vi "UMLEditor_SetMouseCursor.vi"(7 "ViRefToActOn":refnum<vi>, 8 "error in (no error)":errorcluster, 11 "CursorType":T1=enum."NS") -> (0 "error out":errorcluster, 3 "AllCursors":refnum<k1>[](array[refnum]))   [LabVIEW 2016]
uses:
  <resource>/Framework/Providers/Open_GDS/UML/UMLEditor/UMLEditor_Cursortype.ctl
  <vilib>/Utility/cursorutil.llb/Set Cursor (Icon Pict).vi
  <vilib>/Utility/cursorutil.llb/Set Cursor (Cursor ID).vi
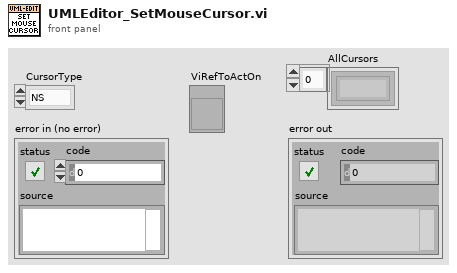
[diagram p1: front panel]
types:
  T1 = typedef "UMLEditor_Cursortype.ctl" = enum16{"Arrow", "Move", "Finger", "Wait", "NS", "WE", "NESW", "NWSE"}
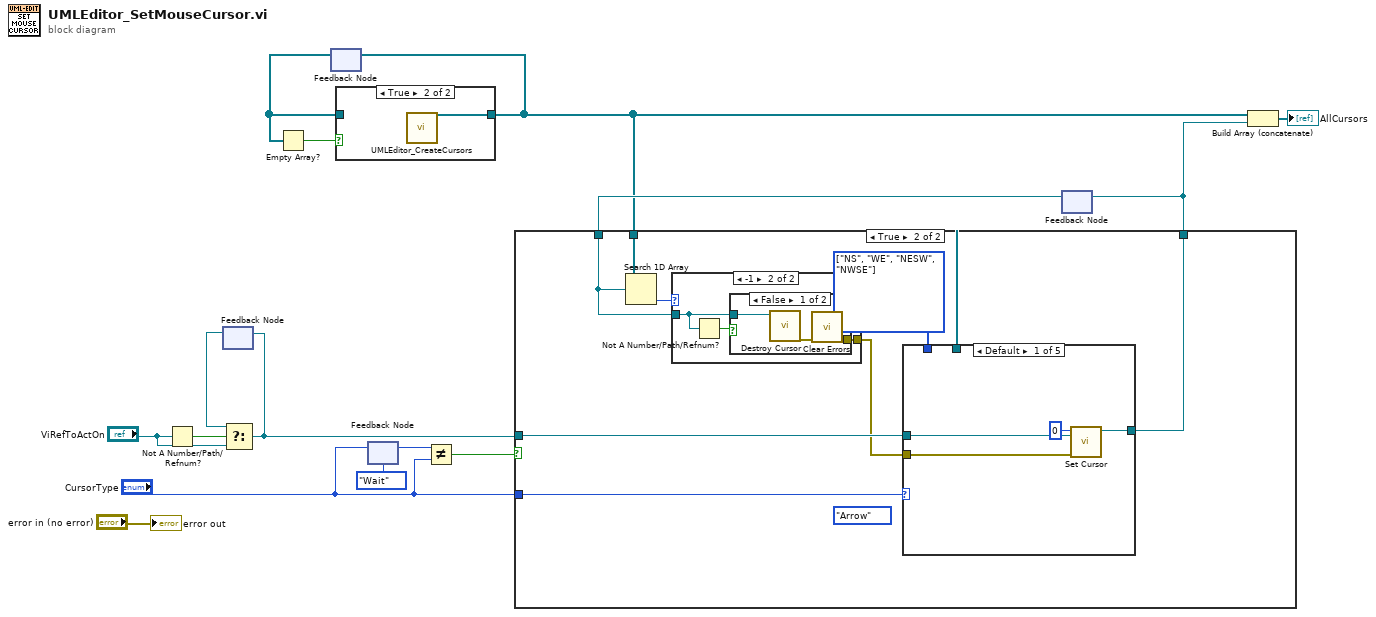
[diagram p0: block diagram]
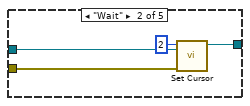
[diagram p3: hidden frame]
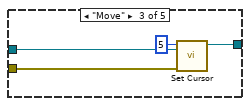
[diagram p4: hidden frame]
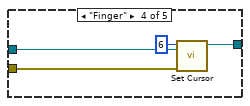
[diagram p5: hidden frame]
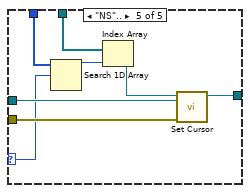
[diagram p6: hidden frame]
diagram:
  n1 = Not A Number/Path/Refnum?(number/path/refnum="ViRefToActOn") -> (NaN/Path/Refnum?=w13:bool)
  n2 = feedback #1() -> (w11:refnum<vi>)  [unwired: 1 in]
  n3 = Select(t=w11, s=w13, f="ViRefToActOn") -> (s? t:f=w10:refnum<vi>)
  n4 = feedback-in #1(w10) -> ()
  n5 = feedback #2() -> (w14:refnum<k1>[])  [unwired: 1 in]
  n6 = Empty Array?(array=w14) -> (empty?=w15:bool)
  n7 = case shown="True" w15 {
    tunnel: w14 -> [w16 _]
    tunnel: [w16 w17] -> w2
    frame False {
    }
    frame True {
      n8 = call <resource>:"UMLEditor_CreateCursors.vi"() -> ("Array"=w17:refnum<k1>[])  [unwired: 10 in, 1 out]
    }
  }
  n9 = feedback-in #2(w2) -> ()
  n10 = feedback #3(UMLEditor_Cursortype."Wait" ("CursorType")) -> (w4:T1)
  n11 = feedback-in #3("CursorType") -> ()
  n12 = Not Equal?(x=w4, y="CursorType") -> (x != y?=w1:bool)
  n13 = feedback #4() -> (w9:refnum<k1>)  [unwired: 1 in]
  n14 = case shown="True" w1 {
    tunnel: w10 -> [_ w26]
    tunnel: w9 -> [w18 w24]
    tunnel: [w18 w21] -> w8
    tunnel: "CursorType" -> [_ w20]
    tunnel: w2 -> [_ w19]
    frame False {
    }
    frame True {
      w22 = T1[] [enum."NS", enum."WE", enum."NESW", enum."NWSE"] items=["Arrow", "Move", "Finger", "Wait", "NS", "WE", "NESW", "NWSE"]
      (unwired) UMLEditor_Cursortype."Arrow" ("CursorType")
      n15 = Search 1D Array(1D array=w19, element=w24) -> (index of element=w23:i32)  [unwired: 1 in]
      n16 = case shown="-1" w23 {
        tunnel: [_ w53] -> w25
        tunnel: w24 -> [_ w52]
        frame 0, Default {
        }
        frame -1 {
          n17 = Not A Number/Path/Refnum?(number/path/refnum=w52) -> (NaN/Path/Refnum?=w51:bool)
          n18 = case shown="False" w51 {
            tunnel: [w55 _] -> w53
            tunnel: w52 -> [w54 _]
            frame False {
              n19 = call <vilib>:"Destroy Cursor.vi"("cursor ID"=w54) -> ("error out"=w56:errorcluster)  [unwired: 9 in]
              n20 = call <vilib>:"Clear Errors.vi"("error in (no error)"=w56) -> ("error out"=w55:errorcluster)  [unwired: 5 in, 1 out]
            }
            frame True {
            }
          }
        }
      }
      n21 = case shown="Default" w20 {
        selector: w20 -> [_ _ _ _ w46]
        tunnel: w26 -> [w30 w34 w38 w42 w50]
        tunnel: [w29 w33 w37 w41 w49] -> w21
        tunnel: w25 -> [w28 w32 w36 w40 w48]
        tunnel: w22 -> [_ _ _ _ w47]
        tunnel: w19 -> [_ _ _ _ w45]
        frame Default {
          n22 = call-poly <vilib>:"Set Cursor.vi"("error in (no error)"=w28, "VI reference (current VI)"=w30, "icon"=u16 0) -> ("previous cursor ID"=w29:refnum<k1>)  [unwired: 8 out]
        }
        frame "Wait" {
          n23 = call-poly <vilib>:"Set Cursor.vi"("error in (no error)"=w32, "VI reference (current VI)"=w34, "icon"=u16 2) -> ("previous cursor ID"=w33:refnum<k1>)  [unwired: 8 out]
        }
        frame "Move" {
          n24 = call-poly <vilib>:"Set Cursor.vi"("error in (no error)"=w36, "VI reference (current VI)"=w38, "icon"=u16 5) -> ("previous cursor ID"=w37:refnum<k1>)  [unwired: 8 out]
        }
        frame "Finger" {
          n25 = call-poly <vilib>:"Set Cursor.vi"("error in (no error)"=w40, "VI reference (current VI)"=w42, "icon"=u16 6) -> ("previous cursor ID"=w41:refnum<k1>)  [unwired: 8 out]
        }
        frame "NS".. {
          n26 = Search 1D Array(1D array=w47, element=w46) -> (index of element=w44:i32)  [unwired: 1 in]
          n27 = Index Array(array=w45, index=w44) -> (element=w43:refnum<k1>)
          n28 = call-poly <vilib>:"Set Cursor.vi"("error in (no error)"=w48, "VI reference (current VI)"=w50, "cursor ID"=w43) -> ("previous cursor ID"=w49:refnum<k1>)  [unwired: 8 out]
        }
      }
    }
  }
  n29 = feedback-in #4(w8) -> ()
  n30 = Build Array (concatenate)(w2, w8) -> (→"AllCursors":refnum<k1>[])
  "error out" <- "error in (no error)"
